vi "Run Inflation.vi"(7 "Main Stop":bool, 8 "error in (no error)":errorcluster, 9 "Test Variables":T1, 10 "PWM Range":cluster{"High PW":dbl, "Low PW":dbl}, 11 "Test Time":dbl) -> (0 "error out":errorcluster, 1 "Camera Framerate":dbl, 2 "Camera Buffer":u32, 3 "Diameter (mm)":dbl, 4 "Stop test?":bool, 5 "Force Data":dbl[](array[numeric]))   [LabVIEW 2020]
uses:
  Controls/Test Variables.ctl
  Controls/Serpoint.ctl
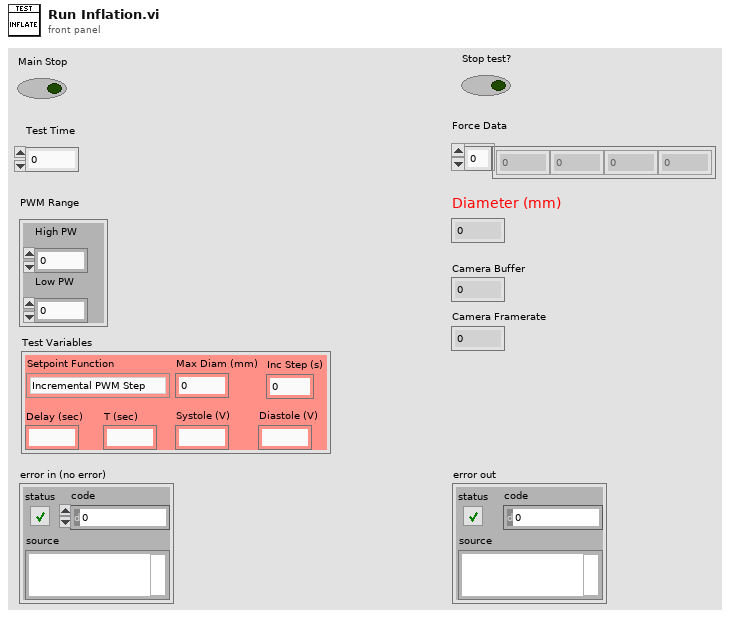
[diagram p1: front panel]
types:
  T1 = typedef "Test Variables.ctl" = cluster{"Setpoint Function":T2, "Max Diam (mm)":dbl, "Delay (sec)":dbl, "T (sec)":dbl, "Diastole (V)":dbl, "Systole (V)":dbl, "Inc Step (s)":dbl}
  T2 = typedef "Serpoint.ctl" = enum16{"Incremental PWM Step", "PWM Step", "Ramp", "Sinusoidal", "Blood-Pressure"}
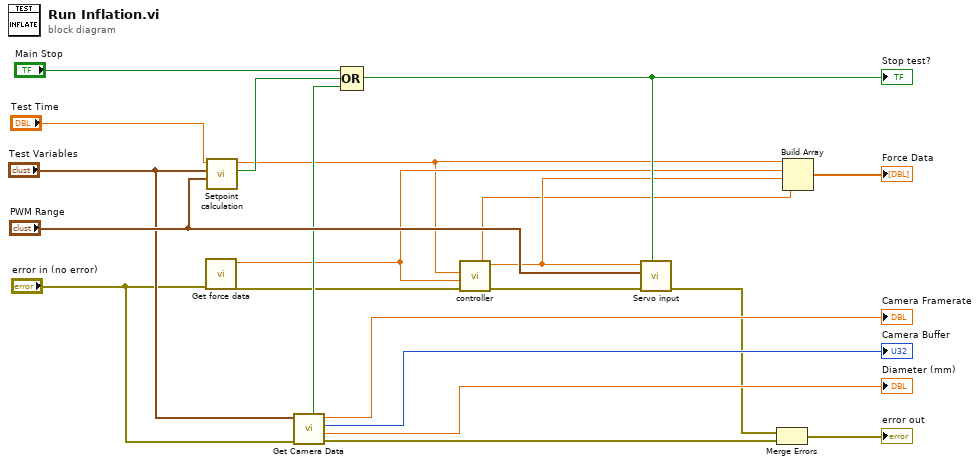
[diagram p0: block diagram]
diagram:
  n1 = call "Get force data.vi"("error in (no error)"="error in (no error)") -> ("error out"=w14:errorcluster, "FS Data"=w5:dbl)  [unwired: 9 in]
  n2 = call "Setpoint calculation.vi"("PWM Range"="PWM Range", "Test Variables"="Test Variables", "Current test time"="Test Time") -> ("Stop?"=w18:bool, "setpoint"=w2:dbl)  [unwired: 7 in]
  n3 = call "Get Camera Data.vi"("error in (no error)"="error in (no error)", "Test Variables"="Test Variables") -> ("error out"=w7:errorcluster, "Diameter (mm)"=→"Diameter (mm)":dbl, "Camera Buffer"=→"Camera Buffer":u32, "Camera Framerate"=→"Camera Framerate":dbl, "Stop?"=w17:bool)  [unwired: 5 in]
  n4 = Compound Arithmetic op=OR("Main Stop", w18, w17) -> (w21:bool)
  "Stop test?" <- w21
  n5 = call "controller.vi"("error in (no error)"=w14, "FS Data"=w5, "Setpoint"=w2) -> ("error out"=w15:errorcluster, "Uncoerced Output"=w3:dbl, "Output"=w4:dbl)  [unwired: 6 in]
  n6 = call "Servo input.vi"("Stop? (F)"=w21, "error in (no error)"=w15, "PWM Range"="PWM Range", "Servo Input"=w4) -> ("error out"=w8:errorcluster)  [unwired: 7 in]
  n7 = Merge Errors(w8, w7) -> (→"error out":errorcluster)
  n8 = Build Array(w2, w5, w4, w3) -> (→"Force Data":dbl[])
